vi "BURST SCPI Driver.vi"(8 "error in (no error)":errorcluster, 11 "VISA resource name":refnum<visa-resource-name>) -> (0 "error out":errorcluster, 2 "read buffer":string)   [LabVIEW 2025]
uses:
  <vilib>/Instr/_visa.llb/VISA Open Access Mode.ctl
  <vilib>/Utility/error.llb/Trim Whitespace One-Sided.vi
  <instrlib>/Agilent U2000 Series/Agilent U2000 Series.lvlib
  3712be93-6b53-4822-bb95-8a507c1bf034.vi
panel:
  in  "Boolean":bool
  in  "write buffer 2":string
  out "write return count 2":u32
  out "Measurement (dBm) 2":dbl
  out "read return count 2":u32
  out "Retries 2":i32
  out "Command 2":string
  in  "OK Button":bool
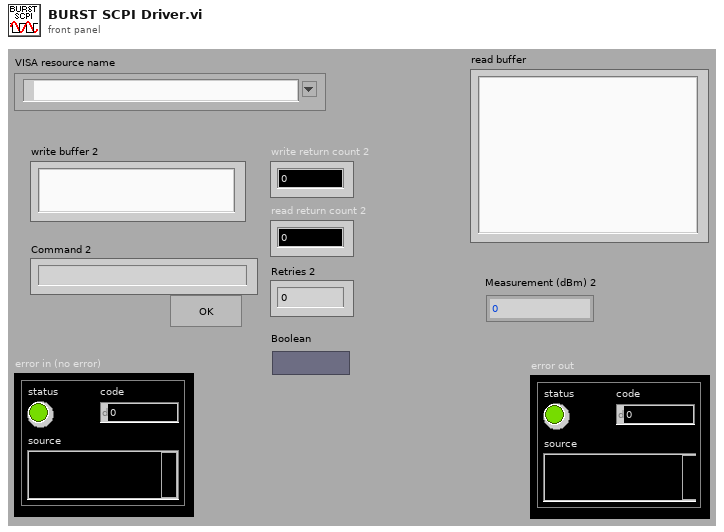
[diagram p1: front panel]
types:
  T1 = typedef "VISA Open Access Mode.ctl" = u32
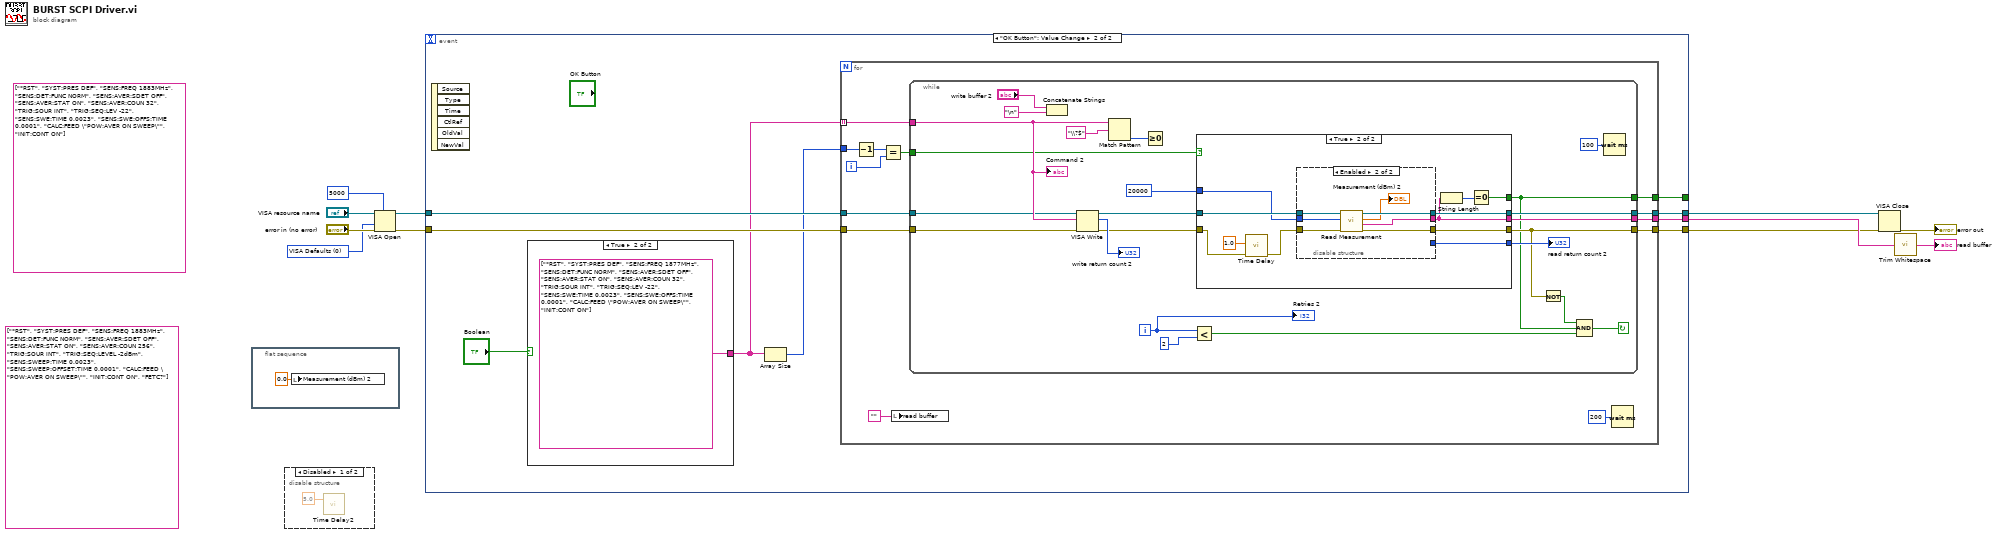
[diagram p0: block diagram]
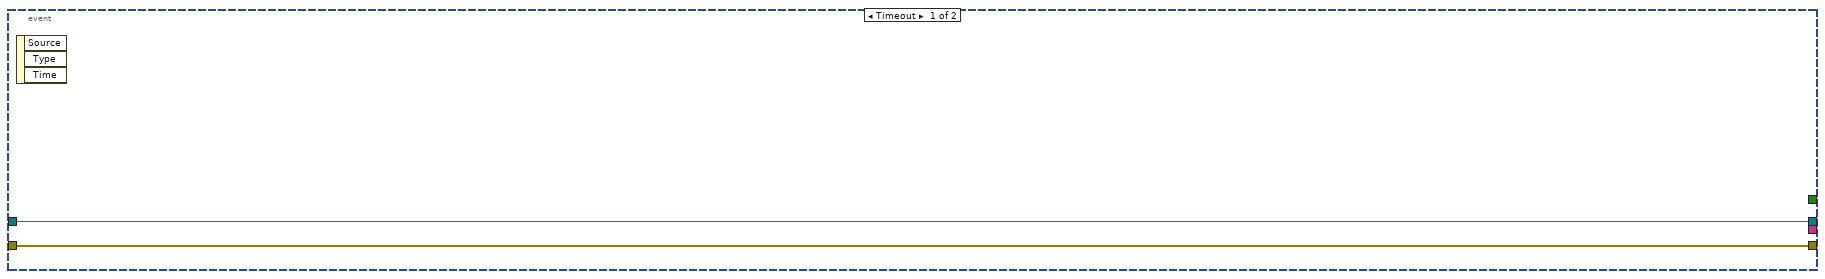
[diagram p2: hidden frame]
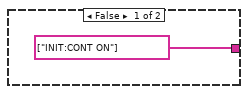
[diagram p3: hidden frame]
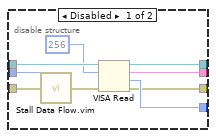
[diagram p5: hidden frame]
diagram:
  (unwired) string[] ["*RST", "SYST:PRES DEF", "SENS:FREQ 1883MHz", "SENS:DET:FUNC NORM", "SENS:AVER:SDET OFF", "SENS:AVER:STAT ON", "SENS:AVER:COUN 32", "TRIG:SOUR INT", "TRIG:SEQ:LEV -22", "SENS:SWE:TIME 0.0023", "SENS:SWE:OFFS:TIME 0.0001", "CALC:FEED \"POW:AVER ON SWEEP\"", "INIT:CONT ON"]
  (unwired) string[] ["*RST", "SYST:PRES DEF", "SENS:FREQ 1883MHz", "SENS:DET:FUNC NORM", "SENS:AVER:SDET OFF", "SENS:AVER:STAT ON", "SENS:AVER:COUN 256", "TRIG:SOUR INT", "TRIG:SEQ:LEVEL -2dBm", "SENS:SWEEP:TIME 0.0023", "SENS:SWEEP:OFFSET:TIME 0.0001", "CALC:FEED \"POW:AVER ON SWEEP\"", "INIT:CONT ON", "FETC?"]
  w5 = T1 0 items=["VISA Defaults"=0, "Exclusive Lock"=1, "Load Configured Settings"=4] ("Access Mode")
  n1 = flat-sequence {
    frame #0 {
      n2 = local write "Measurement (dBm) 2"(0.0 ("Measurement (dBm)")) -> ()
    }
  }
  n3 = disable-structure shown="Disabled" {
    frame Disabled {
      n4 = call "Time Delay2"("Delay Time (s)"=5.0) -> ()  [unwired: 10 in, 1 out]
    }
    frame Enabled {
    }
  }
  n5 = VISA Open(timeout (0)=u32 5000 ("VISA Open timeout (0)"), access mode=w5, error in (no error)="error in (no error)", VISA resource name="VISA resource name") -> (VISA resource name=w3:refnum<visa-resource-name>, error out=w4:errorcluster)  [unwired: 1 in]
  n6 = event shown="[1] \"OK Button\": Value Change" {
    selector: _ -> [_ _]
    dyn-events: _ -> [_ _]
    timeout: _ -> [_ _]
    tunnel: [_ w24] -> w2
    tunnel: [w14 w23] -> w1
    tunnel: [_ w22] -> _
    tunnel: [w15 w21] -> w9
    tunnel: w4 -> [w14 w20]
    tunnel: w3 -> [w15 w19]
    event Timeout {
      n7 = event-data() -> ()  [unwired: 1 in, 3 out]
    }
    event "OK Button": Value Change {
      n8 = event-data() -> ()  [unwired: 1 in, 6 out]
      n9 = case shown="True" "Boolean" {
        tunnel: [string[] ["INIT:CONT ON"] string[] ["*RST", "SYST:PRES DEF", "SENS:FREQ 1877MHz", "SENS:DET:FUNC NORM", "SENS:AVER:SDET OFF", "SENS:AVER:STAT ON", "SENS:AVER:COUN 32", "TRIG:SOUR INT", "TRIG:SEQ:LEV -22", "SENS:SWE:TIME 0.0023", "SENS:SWE:OFFS:TIME 0.0001", "CALC:FEED \"POW:AVER ON SWEEP\"", "INIT:CONT ON"]] -> w17
        frame False {
        }
        frame True {
        }
      }
      n10 = Array Size(array=w17) -> (size(s)=w18:i32)
      n11 = for {
        tunnel: w17 -> [w39] mode=indexing
        tunnel: [w36] -> w24
        tunnel: [w35] -> w23
        tunnel: [w34] -> w22
        tunnel: [w33] -> w21
        tunnel: w20 -> [w32]
        tunnel: w19 -> [w31]
        tunnel: w18 -> [w27]
        i -> [w30]
        n12 = Decrement(x=w27) -> (x-1=w28:i32)
        n13 = Equal?(x=w28, y=w30) -> (x = y?=w29:bool)
        n14 = local write "read buffer"("") -> ()
        n15 = while {
          tunnel: [w46] -> w35
          tunnel: [w44] -> w34
          tunnel: [w56] -> w33
          tunnel: [w53] -> w36
          tunnel: w39 -> [w48]
          tunnel: w32 -> [w40]
          tunnel: w31 -> [w47]
          tunnel: w29 -> [w41]
          i -> [w51]
          stop <- w42 continue-if-true
          n16 = Concatenate Strings("write buffer 2", "\n") -> ()  [unwired: 1 out]
          n17 = VISA Write(VISA resource name=w47, write buffer=w48, error in (no error)=w40) -> (VISA resource name out=w57:refnum<visa-resource-name>, return count=→"write return count 2":u32, error out=w54:errorcluster)
          n18 = Match Pattern(string=w48, regular expression="\\?$") -> (offset past match=w59:i32)  [unwired: 1 in, 3 out]
          n19 = Greater Or Equal To 0?(x=w59) -> ()  [unwired: 1 out]
          n20 = Less?(x=w51, y=2) -> (x < y?=w43:bool)
          n21 = case shown="True" w41 {
            tunnel: w57 -> [w64 w75]
            tunnel: w54 -> [w63 w66]
            tunnel: [w64 w74] -> w56
            tunnel: [_ w69] -> w53
            tunnel: [_ w73] -> w52
            tunnel: [w63 w72] -> w46
            tunnel: [_ w71] -> w44
            tunnel: u32 20000 ("milliseconds to wait") -> [_ w70]
            frame False {
            }
            frame True {
              n22 = call "Time Delay"("error in (no error)"=w66, "Delay Time (s)"=1.0) -> ("error out"=w65:errorcluster)  [unwired: 9 in]
              n23 = disable-structure shown="Enabled" {
                disable-tunnel: w75 -> [w84 w90]
                disable-tunnel: [w83 w89] -> w74
                disable-tunnel: [w82 w86] -> w69
                disable-tunnel: [w81 _] -> w73
                disable-tunnel: [w80 w87] -> w72
                disable-tunnel: w65 -> [w79 w88]
                disable-tunnel: w70 -> [w76 w91]
                frame Disabled {
                  n24 = call "Stall Data Flow.vim"("value in"=w79, "milliseconds to wait"=w76) -> ("value out"=w77:errorcluster)  [unwired: 1 out]
                  n25 = VISA Read(VISA resource name=w84, byte count=u32 256, error in (no error)=w77) -> (VISA resource name out=w83:refnum<visa-resource-name>, read buffer=w82:string, return count=w81:u32, error out=w80:errorcluster)
                }
                frame Enabled {
                  n26 = call <instrlib>:"Read Measurement.vi"("error in (no error)"=w88, "Timeout (10000 ms)"=w91, "VISA resource name"=w90) -> ("error out"=w87:errorcluster, "read buffer"=w86:string, "Measurement"=→"Measurement (dBm) 2":dbl, "VISA resource name out"=w89:refnum<visa-resource-name>)  [unwired: 5 in]
                }
              }
              n27 = String Length(string=w69) -> (length=w68:i32)
              n28 = Equal To 0?(x=w68) -> (x = 0?=w71:bool)
            }
          }
          "read return count 2" <- w52
          n29 = Not(x=w46) -> (.not. x?=w45:bool)
          n30 = Compound Arithmetic op=AND(w45, w44, w43) -> (w42:bool)
          n31 = Wait (ms)(milliseconds to wait=u32 100) -> ()  [unwired: 1 out]
          "Retries 2" <- w51
          "Command 2" <- w48
        }
        n32 = Wait (ms)(milliseconds to wait=u32 200) -> ()  [unwired: 1 out]
      }
    }
  }
  n33 = VISA Close(VISA resource name=w9, error in (no error)=w1) -> (error out=→"error out":errorcluster)
  n34 = call <vilib>:"Trim Whitespace.vi"("string"=w2) -> ("trimmed string"=→"read buffer":string)  [unwired: 1 in]
